vi "Tree Finding Specific Item Symbol Tag.vi"(6 "Symbol Index Array In":i32[](array[numeric]), 8 "Tags In":string[](array[string]), 9 "Tag In":string, 11 "Selection Tree In":refnum<vi>) -> (0 "Tags Out":string[](array[string]), 3 "Selection Tree Out":refnum<vi>)   [LabVIEW 2024]
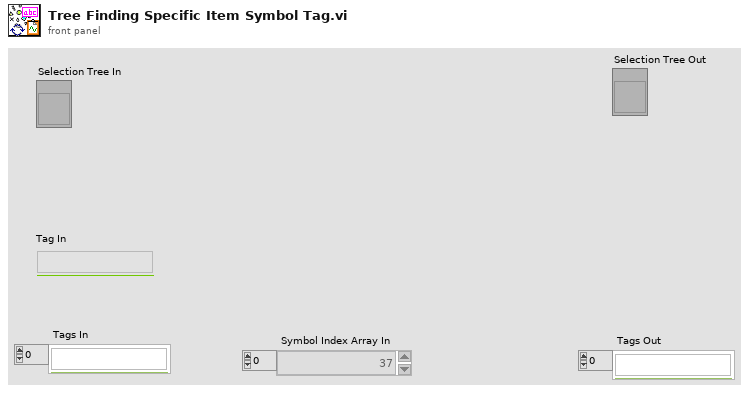
[diagram p1: front panel]
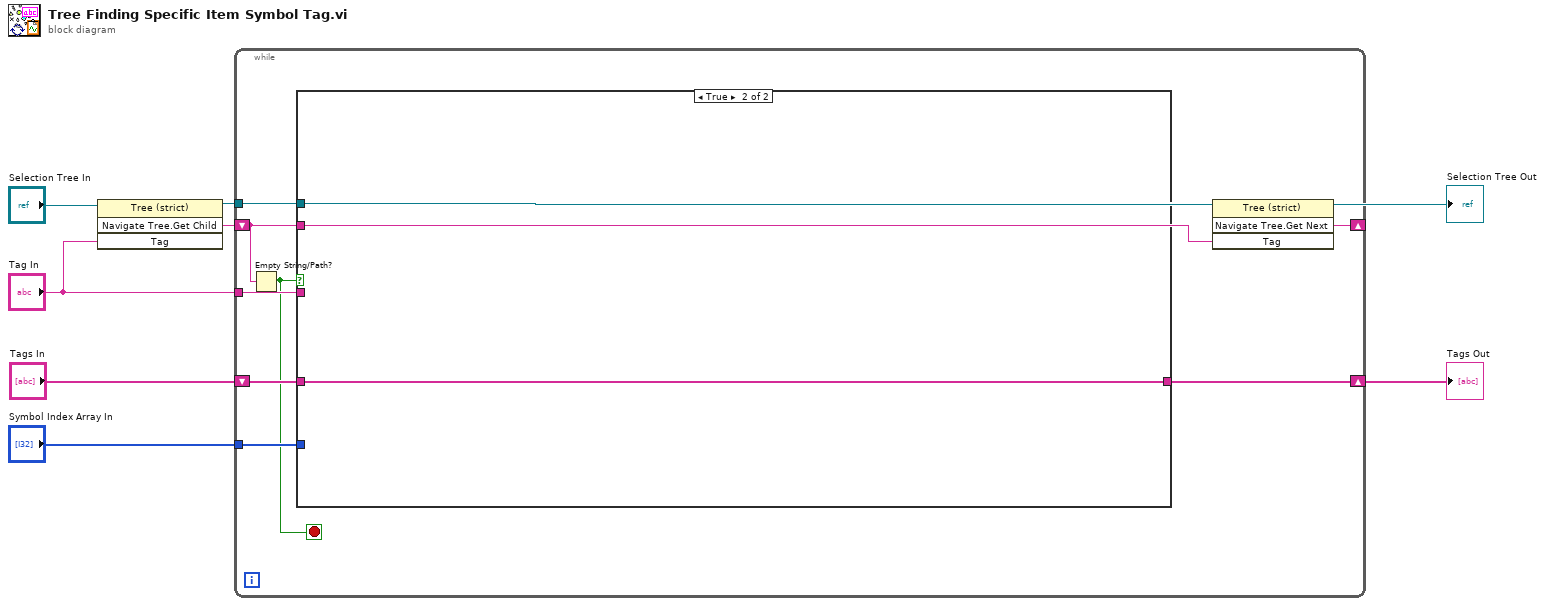
[diagram p0: block diagram]
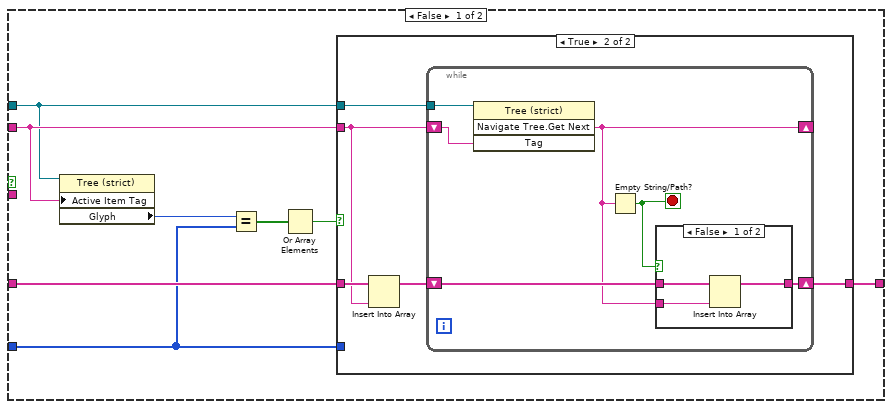
[diagram p2: hidden frame]
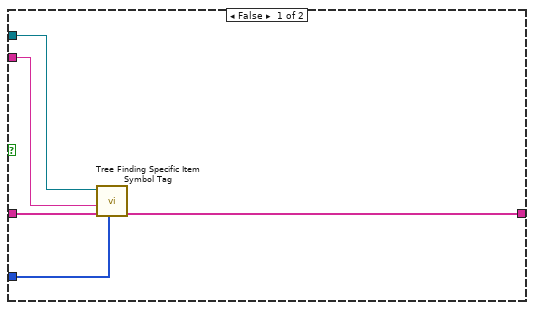
[diagram p3: hidden frame]
diagram:
  n1 = invoke class="Tree (strict)" method="Navigate Tree.Get Child"(reference="Selection Tree In", "Tag"="Tag In") -> (reference out=w4:refnum<vi>, "Navigate Tree:Get Child"=w5:string)  [unwired: 2 in, 2 out]
  "Selection Tree Out" <- w4
  n2 = while {
    tunnel: "Tag In" -> [w15]
    tunnel: w4 -> [w8]
    tunnel: "Symbol Index Array In" -> [w12]
    shift-right: [w13] -> w2
    shift-left: "Tags In" -> [w14]
    shift-right: [w10] -> _
    shift-left: w5 -> [w9]
    stop <- w11 stop-if-true
    n3 = Empty String/Path?(string/path=w9) -> (empty?=w11:bool)
    n4 = case shown="True" w11 {
      tunnel: w15 -> [_ _]
      tunnel: w9 -> [w22 _]
      tunnel: w8 -> [w21 _]
      tunnel: w14 -> [w20 w44]
      tunnel: [w19 w44] -> w13
      tunnel: w12 -> [w16 _]
      frame False {
        n5 = property class="Tree (strict)"(reference=w21, "Active Item Tag"=w22) -> ("Glyph"=w23:i32)  [unwired: 1 in, 2 out]
        n6 = Equal?(x=w23, y=w16) -> (x = y?=w17:bool[])
        n7 = Or Array Elements(Boolean array=w17) -> (logical OR=w18:bool)
        n8 = case shown="True" w18 {
          tunnel: w22 -> [w26 w30]
          tunnel: w21 -> [w25 w29]
          tunnel: w20 -> [w28 w33]
          tunnel: [w27 w31] -> w19
          tunnel: w16 -> [w24 _]
          frame False {
            n9 = call "Tree Finding Specific Item Symbol Tag.vi"("Symbol Index Array In"=w24, "Tags In"=w28, "Tag In"=w26, "Selection Tree In"=w25) -> ("Tags Out"=w27:string[])  [unwired: 6 in, 1 out]
          }
          frame True {
            n10 = Insert Into Array(array=w33, new element=w30) -> (w32:string[])  [unwired: 1 in]
            n11 = while {
              shift-right: [w35] -> w31
              shift-left: w32 -> [w36]
              shift-right: [w34] -> _
              shift-left: w30 -> [w38]
              tunnel: w29 -> [w39]
              stop <- w37 stop-if-true
              n12 = invoke class="Tree (strict)" method="Navigate Tree.Get Next"(reference=w39, "Tag"=w38) -> ("Navigate Tree:Get Next Item"=w34:string)  [unwired: 2 in, 3 out]
              n13 = Empty String/Path?(string/path=w34) -> (empty?=w37:bool)
              n14 = case shown="False" w37 {
                tunnel: w36 -> [w42 w43]
                tunnel: [w41 w43] -> w35
                tunnel: w34 -> [w40 _]
                frame False {
                  n15 = Insert Into Array(array=w42, new element=w40) -> (w41:string[])  [unwired: 1 in]
                }
                frame True {
                }
              }
            }
          }
        }
      }
      frame True {
      }
    }
    n16 = invoke class="Tree (strict)" method="Navigate Tree.Get Next"(reference=w8, "Tag"=w9) -> ("Navigate Tree:Get Next Item"=w10:string)  [unwired: 2 in, 3 out]
  }
  "Tags Out" <- w2
